vi "cluster2array.vi"(1 "temp data":cluster{dbl[][]}[](array[cluster])) -> (0 "temp data array":dbl[][][](array[numeric]))   [LabVIEW 2013]
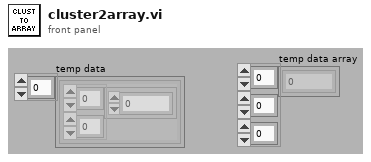
[diagram p1: front panel]
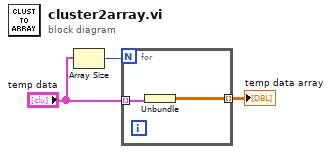
[diagram p0: block diagram]
diagram:
  n1 = Array Size(array="temp data") -> (size(s)=w2:i32)
  n2 = for {
    N: w2 -> [_]
    tunnel: "temp data" -> [w5] mode=indexing
    tunnel: [w4] -> w1 mode=indexing
    n3 = Unbundle(w5) -> (w4:dbl[][])
  }
  "temp data array" <- w1
